vi "FGV_EventToScreens.vi"(7 "Command":T1, 8 "error in (no error)":errorcluster) -> (0 "error out":errorcluster, 3 "To Screens Event":refnum<user-event>)   [LabVIEW 2011]
uses:
  EnumFgvEventCommand.ctl
  ToScreen.ctl
  ToScreensCommand.ctl
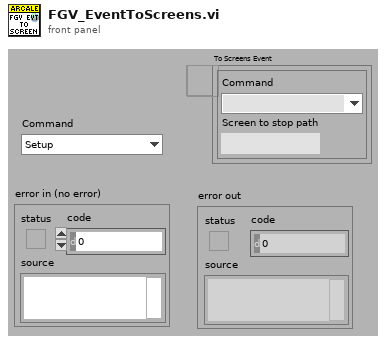
[diagram p1: front panel]
types:
  T1 = typedef "EnumFgvEventCommand.ctl" = enum16{"Setup", "Cleanup", "Get"}
  T2 = typedef "ToScreen.ctl" = cluster{"Command":T3, "Screen to stop path":path}
  T3 = typedef "ToScreensCommand.ctl" = enum16{"Stop screen", "Stop all screens"}
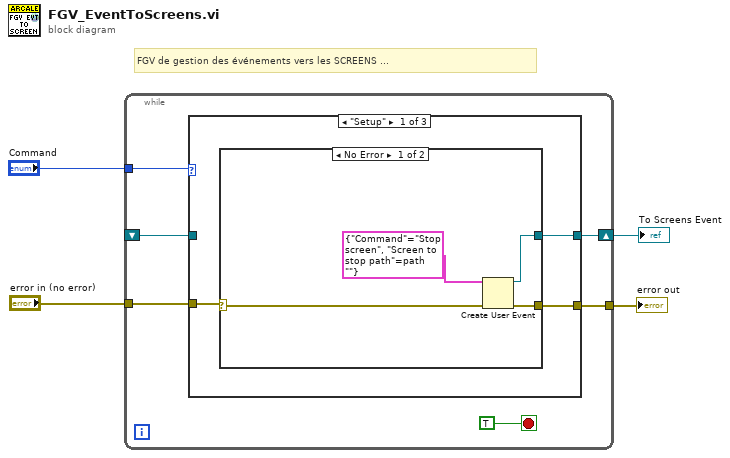
[diagram p0: block diagram]
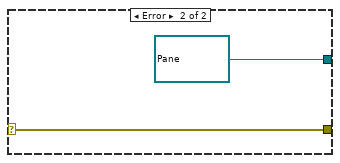
[diagram p2: hidden frame]
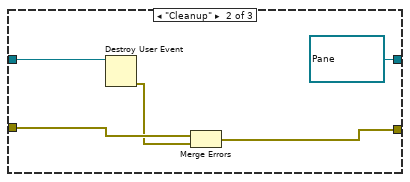
[diagram p3: hidden frame]
diagram:
  # "FGV de gestion des événements vers les SCREENS ..."
  n1 = while {
    tunnel: "error in (no error)" -> [w8]
    tunnel: "Command" -> [w9]
    tunnel: [w7] -> w2
    shift-right: [w6] -> w1
    shift-left: _ -> [w5]
    stop <- TRUE stop-if-true
    n2 = case shown="\"Setup\"" w9 {
      tunnel: w8 -> [w13 w23 w25]
      tunnel: [w12 w22 w25] -> w7
      tunnel: [w11 refnum<user-event> refnum ("To Screens Event") w26] -> w6
      tunnel: w5 -> [_ w24 w26]
      frame "Setup" {
        n3 = case shown="No Error" w13 {
          selector: w13 -> [w17 w19]
          tunnel: [w15 w19] -> w12
          tunnel: [w14 refnum<user-event> refnum ("To Screens Event")] -> w11
          frame No Error {
            n4 = Create User Event(user event datatype=T2 {"Command"=enum."Stop screen", "Screen to stop path"=path ""} ("To Screens Event"), error in=w17) -> (user event=w14:refnum<user-event>, error out=w15:errorcluster)
          }
          frame Error {
          }
        }
      }
      frame "Cleanup" {
        n5 = Destroy User Event(user event=w24) -> (error out=w21:errorcluster)  [unwired: 1 in]
        n6 = Merge Errors(w23, w21) -> (w22:errorcluster)
      }
      frame "Get" {
      }
    }
  }
  "error out" <- w2
  "To Screens Event" <- w1
